vi "Get Image 1 Path.vi"(11 "Image File Type":T1) -> (3 "Image 1 Path out":path)   [LabVIEW 2014]
uses:
  Image Type.ctl
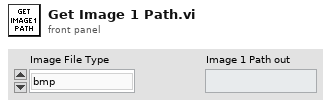
[diagram p1: front panel]
types:
  T1 = typedef "Image Type.ctl" = enum16{"bmp", "jpg", "png"}
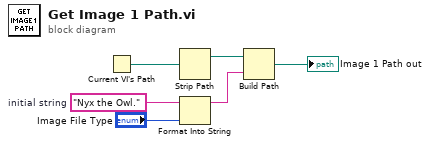
[diagram p0: block diagram]
diagram:
  w5 = "Nyx the Owl."  # initial string
  n1 = Current VI's Path() -> (path=w4:path)
  n2 = Strip Path(path=w4) -> (stripped path=w3:path)  [unwired: 1 out]
  n3 = Format Into String(initial string=w5, "Image File Type") -> (resulting string=w2:string)  [unwired: 2 in, 1 out]
  n4 = Build Path(base path=w3, name or relative path=w2) -> (appended path=→"Image 1 Path out":path)
